vi "RP Save Data.vi"(4 "Signal bits":i32=14, 5 "I-V avg":i32=480, 6 "Mode":T2=enum."Digitizer", 7 "Root Data Folder":path=path "C:/Data", 8 "Error In":errorcluster, 9 "Parameters":T1={"Ranges"=[20.0, 20.0], "Output frequency 1"=50000.0, "Output frequency 2"=50000.0, "Pre-trigger samples"=-100000, "Post-trigger samples"=11534336, "Desimation rate"=125, "Delayed start"=571428} {"Delayed start" format="0x%x (%d)"; "Post-trigger samples" format="0x%x (%d)"; "Pre-trigger samples" format="0x%x (%d)"; "Output frequency 2" format="%#_6p"; "Output frequency 1" format="%#_6p"; "Ranges" format="%#_12p"}, 10 "Data stream":string, 11 "connection ID":refnum<k5>) -> (0 "Error Out":errorcluster, 1 "Channel names":string[](array[string]), 2 "Data File  Path":path, 3 "connection ID out":refnum<k5>)   [LabVIEW 2016]
uses:
  Mode.ctl
  Red Pitaya Parameters.ctl
  File/Controls/File formats.ctl
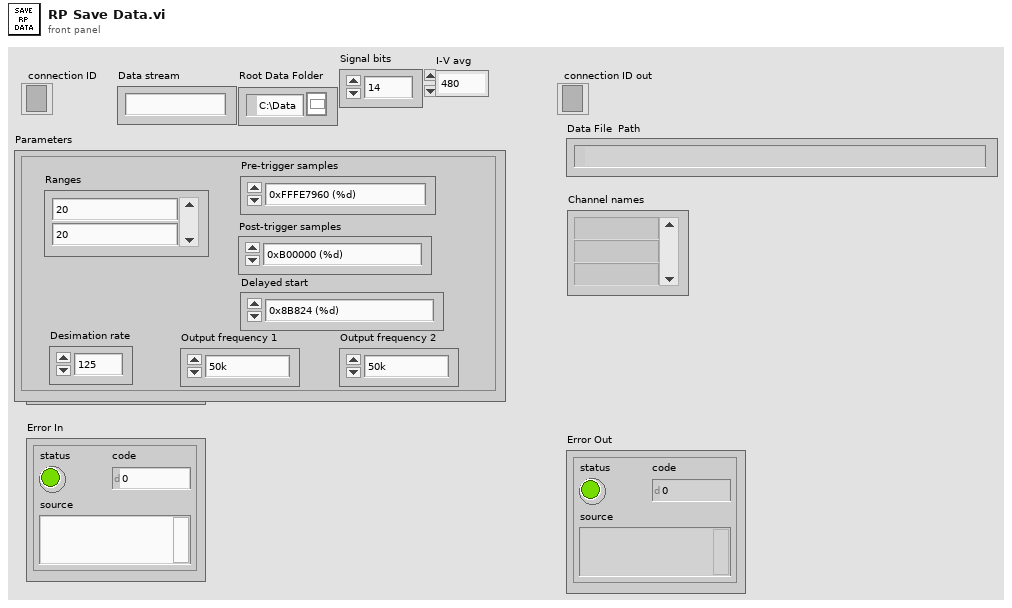
[diagram p1: front panel]
types:
  T1 = typedef "Red Pitaya Parameters.ctl" = cluster{"Ranges":dbl[], "Output frequency 1":dbl, "Output frequency 2":dbl, "Pre-trigger samples":i32, "Post-trigger samples":u64, "Desimation rate":u64, "Delayed start":u64}
  T2 = typedef "Mode.ctl" = enum16{"Filter", "Lockin test", "Snapshot test", "Digitizer", "Current-Voltage"}
  T3 = typedef "File formats.ctl" = enum16{"TDMS", "ASCII", "BINARY"}
  T4 = typedef "RP info.ctl" = cluster{"Range":dbl, "Name":string, "waveform period":dbl, "waveform start":dbl, "Frequency":u32, "Phase":u32}
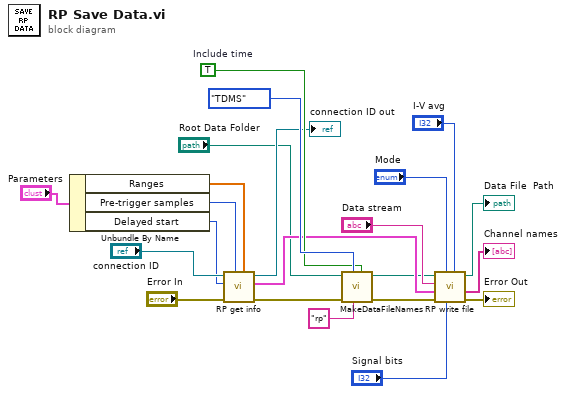
[diagram p0: block diagram]
diagram:
  w20 = TRUE  # Include time
  n1 = Unbundle By Name("Parameters") -> ("Ranges"=w13:dbl[], "Pre-trigger samples"=w12:i32, "Delayed start"=w2:u64)
  n2 = call "RP get info.vi"("Ranges"=w13, "Trigger offset"=w12, "Error In"="Error In", "Delayed start"=w2, "connection ID"="connection ID") -> ("Error Out"=w18:errorcluster, "Channel info"=w17:T4[], "connection ID out"=→"connection ID out":refnum<k5>)  [unwired: 4 in]
  n3 = call "MakeDataFileNames.vi"("Include time"=w20, "File Prefix"="rp", "File format"=File_formats."TDMS", "Error In"=w18, "Root Data Folder"="Root Data Folder") -> ("Error Out"=w19:errorcluster, "Data File  Path"=w4:path)  [unwired: 3 in, 2 out]
  n4 = call "RP write file.vi"("I-V avg"="I-V avg", "Signal bits"="Signal bits", "Mode"="Mode", "Error In"=w19, "Channel info"=w17, "Data"="Data stream", "File Path"=w4) -> ("Error Out"=→"Error Out":errorcluster, "Channel names"=→"Channel names":string[], "File  path out"=→"Data File  Path":path)  [unwired: 2 in]
